vi "Read Power Factor Limits.vi"(0 "VISA resource name":refnum<visa-resource-name>, 11 "error in (no error)":errorcluster) -> (4 "VISA resource name out":refnum<visa-resource-name>, 6 "Power Factor High Limit":dbl, 8 "Power Factor Low Limit":dbl, 15 "error out":errorcluster)   [LabVIEW 2016, in "APT 300XAC Series.lvlib"]
doc: "Reads the power factor limits configured in the power source instrument.\n\nNote : Should be used in program mode only."
uses:
  APT 300XAC Series.lvlib
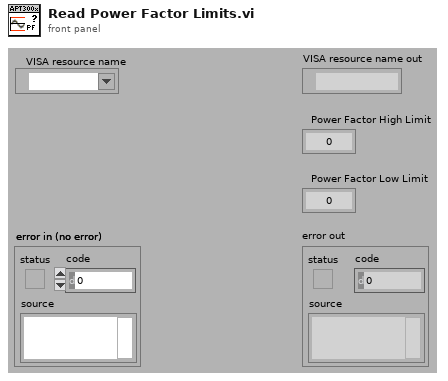
[diagram p1: front panel]
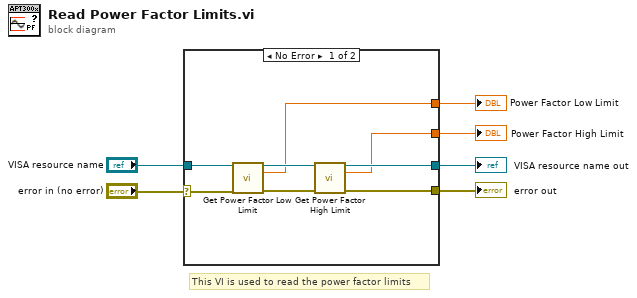
[diagram p0: block diagram]
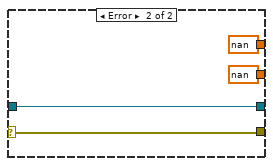
[diagram p2: hidden frame]
diagram:
  # "This VI is used to read the power factor limits"
  n1 = case shown="No Error" "error in (no error)" {
    selector: "error in (no error)" -> [w14 w17]
    tunnel: [w12 w17] -> w5
    tunnel: [w11 w18] -> w4
    tunnel: "VISA resource name" -> [w9 w18]
    tunnel: [w8 nan ("Voltage Low Limit")] -> w2
    tunnel: [w7 nan ("Voltage Low Limit")] -> w1
    frame No Error {
      n2 = call "Get Power Factor Low Limit.vi"("VISA resource name"=w9, "error in (no error)"=w14) -> ("VISA resource name out"=w10:refnum<visa-resource-name>, "Power Factor Low Limit"=w8:dbl, "error out"=w13:errorcluster)  [unwired: 11 in]
      n3 = call "Get Power Factor High Limit.vi"("VISA resource name"=w10, "error in (no error)"=w13) -> ("VISA resource name out"=w11:refnum<visa-resource-name>, "Power Factor High Limit"=w7:dbl, "error out"=w12:errorcluster)  [unwired: 11 in]
    }
    frame Error {
    }
  }
  "error out" <- w5
  "VISA resource name out" <- w4
  "Power Factor High Limit" <- w1
  "Power Factor Low Limit" <- w2
